vi "Main.vi"(11 "Module Admin":refnum<class "Delacor_lib_QMH_Module Admin.lvclass">) -> ()   [LabVIEW 2021, in "Host Interpreter.lvlib"]
doc: "This template is based off of the Queued Message Handler design pattern and the Queued Message Handler project template that ships with LabVIEW.\n\nThe main difference is that the queue is private to this module and communication between modules is performed via Broadcast and Request events.\n\nRequest events are wrapped in public API methods and are handled in the Event Handling Loop (EHL) of this VI. Any module can register for Broadcast events sent by this module. The EHL generates messages based on user interface actions.\n\nThe Message Handling Loop (MHL) processes messages generated by the EHL, or by other messages. The messages are string values, so new messages can be added easily to the Message Cases case structure in the MHL. Each message cluster can also provide an optional value for Message Data, which is a variant that can be converted to whatever message-specific data is required.\n_____\nBased on DQMH Dev Tools: Project Template 7.1.2.1547."
uses:
  Host Interpreter.lvlib
  <vilib>/Delacor/Delacor QMH/Libraries/Module Admin_class/Delacor_lib_QMH_Module Admin.lvclass
  Module Data--cluster.ctl
  Host Initialization--cluster.ctl
  Read Messages from Target HL--cluster.ctl
  Stop Argument--cluster.ctl
  <vilib>/Delacor/Delacor QMH/Libraries/Message Queue_class/Delacor_lib_QMH_Message Queue.lvclass/Delacor_lib_QMH_Message Queue.ctl
  <vilib>/Delacor/Delacor QMH/Libraries/Module Admin_class/Delacor_lib_QMH_Module Admin.lvclass/Delacor_lib_QMH_Module Admin.ctl
  Open UDP Argument--cluster.ctl
  Send Message to Target Argument--cluster.ctl
  Libraries/UDP Comms/UDP Message--cluster.ctl
  Close UDP Argument--cluster.ctl
  Disconnect from Target Argument--cluster.ctl
  Connected to Target Argument--cluster.ctl
  Disconnected from Target Argument--cluster.ctl
  <vilib>/Utility/miscctls.llb/LVPointTypeDef.ctl
  cda96e32-a3c6-4f37-bbf6-85d7dab5b00d.vi
  b5302b80-1133-4ea9-a211-fc2c65372a7a.vi
  1aab31dc-b2c4-46e6-995f-f9a1faaff8ea.vi
  <vilib>/Delacor/Delacor QMH/Libraries/Message Queue_class/Delacor_lib_QMH_Enqueue Message (Single).vi
  <vilib>/Delacor/Delacor QMH/Libraries/Module Admin_class/Delacor_lib_QMH_Get External Launch.vi
  <vilib>/JDP Science/JSONtext/JSON text to Variant.vi
  <vilib>/JDP Science/JSONtext/LVClass Serializer/JSONtext LVClass Serializer.lvclass
  <vilib>/Delacor/Delacor QMH/Libraries/Message Queue_class/Delacor_lib_QMH_Message Queue.lvclass
  Libraries/UDP Comms/UDP Comms.lvlib
  Libraries/Utilities/Utilities.lvlib
  Main HMI/Main HMI.lvlib
panel:
  out "error out":errorcluster
  out "Status":string
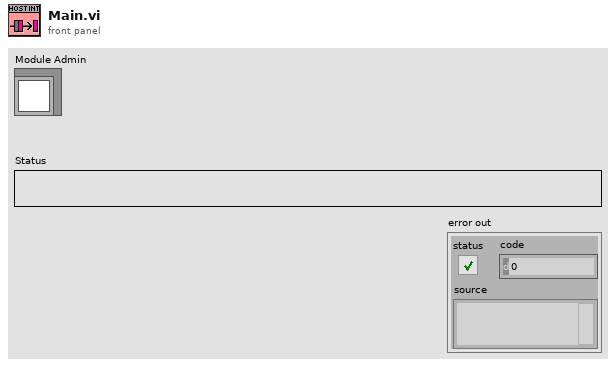
[diagram p1: front panel]
types:
  T1 = typedef "Host Interpreter.lvlib/Request Events--cluster.ctl" = cluster{"Stop Module":refnum<user-event>, "Show Panel":refnum<user-event>, "Hide Panel":refnum<user-event>, "Get Module Execution Status":refnum<user-event>, "Show Diagram":refnum<user-event>, "Connect to Target":refnum<user-event>, "Private.Get Config":refnum<user-event>, "Private.Open UDP":refnum<user-event>, "Private.Start Reading MSGs":refnum<user-event>, "Private.Send Message to Target":refnum<user-event>, "Request Connections to Target":refnum<user-event>, "Private.Close UDP":refnum<user-event>, "Update Polling Time":refnum<user-event>, "Disconnect from Target":refnum<user-event>, "Private.Connected to Target":refnum<user-event>, "Private.Disconnected from Target":refnum<user-event>}
  T2 = typedef "Host Interpreter.lvlib/Read Messages from Target HL--cluster.ctl" = cluster{"Host UDP connection ref":refnum<k16>, "Target IP":string, "Target UDP Listening Port":u16}
  T3 = typedef "Host Interpreter.lvlib/Module Data--cluster.ctl" = cluster{"Status":string, "Host UDP connection ref":refnum<k16>, "Target IP":string, "Target UDP Listening Port":u16, "Host Config":T4, "Polling Rate (ms)":i32, "UDP Connected?":bool, "Connected to Target?":bool}
  T4 = typedef "UDP Comms.lvlib/Host Initialization--cluster.ctl" = cluster{"Host IP":string, "Host Listening Port":u16, "MasterHost?":bool}
  T5 = enum32{"invalid lock state", "Not Locked", "Locked (No Password)", "Password-protected"}
  T6 = typedef "Host Interpreter.lvlib/Stop Argument--cluster.ctl" = cluster{"Origin":string, "Exit via Stop Module Req?":bool, "Wait for Module to stop?":bool}
  T7 = typedef "Host Interpreter.lvlib/Open UDP Argument--cluster.ctl" = cluster{"Boolean":bool}
  T8 = typedef "Host Interpreter.lvlib/Send Message to Target Argument--cluster.ctl" = cluster{"First Message?":bool, "UDP Message":T9}
  T9 = typedef "UDP Comms.lvlib/UDP Message--cluster.ctl" = cluster{"Command":string, "Data":variant}
  T10 = typedef "Host Interpreter.lvlib/Close UDP Argument--cluster.ctl" = cluster{"Boolean":bool}
  T11 = typedef "Host Interpreter.lvlib/Disconnect from Target Argument--cluster.ctl" = cluster{"Boolean":bool}
  T12 = typedef "Host Interpreter.lvlib/Connected to Target Argument--cluster.ctl" = cluster{"Boolean":bool}
  T13 = typedef "Host Interpreter.lvlib/Disconnected from Target Argument--cluster.ctl" = cluster{"Boolean":bool}
  T14 = typedef "LVPointTypeDef.ctl" = cluster{"Horizontal":i16, "Vertical":i16}
  T15 = enum32{"Invalid", "Standard", "Closed", "Hidden", "Minimized", "Maximized"}
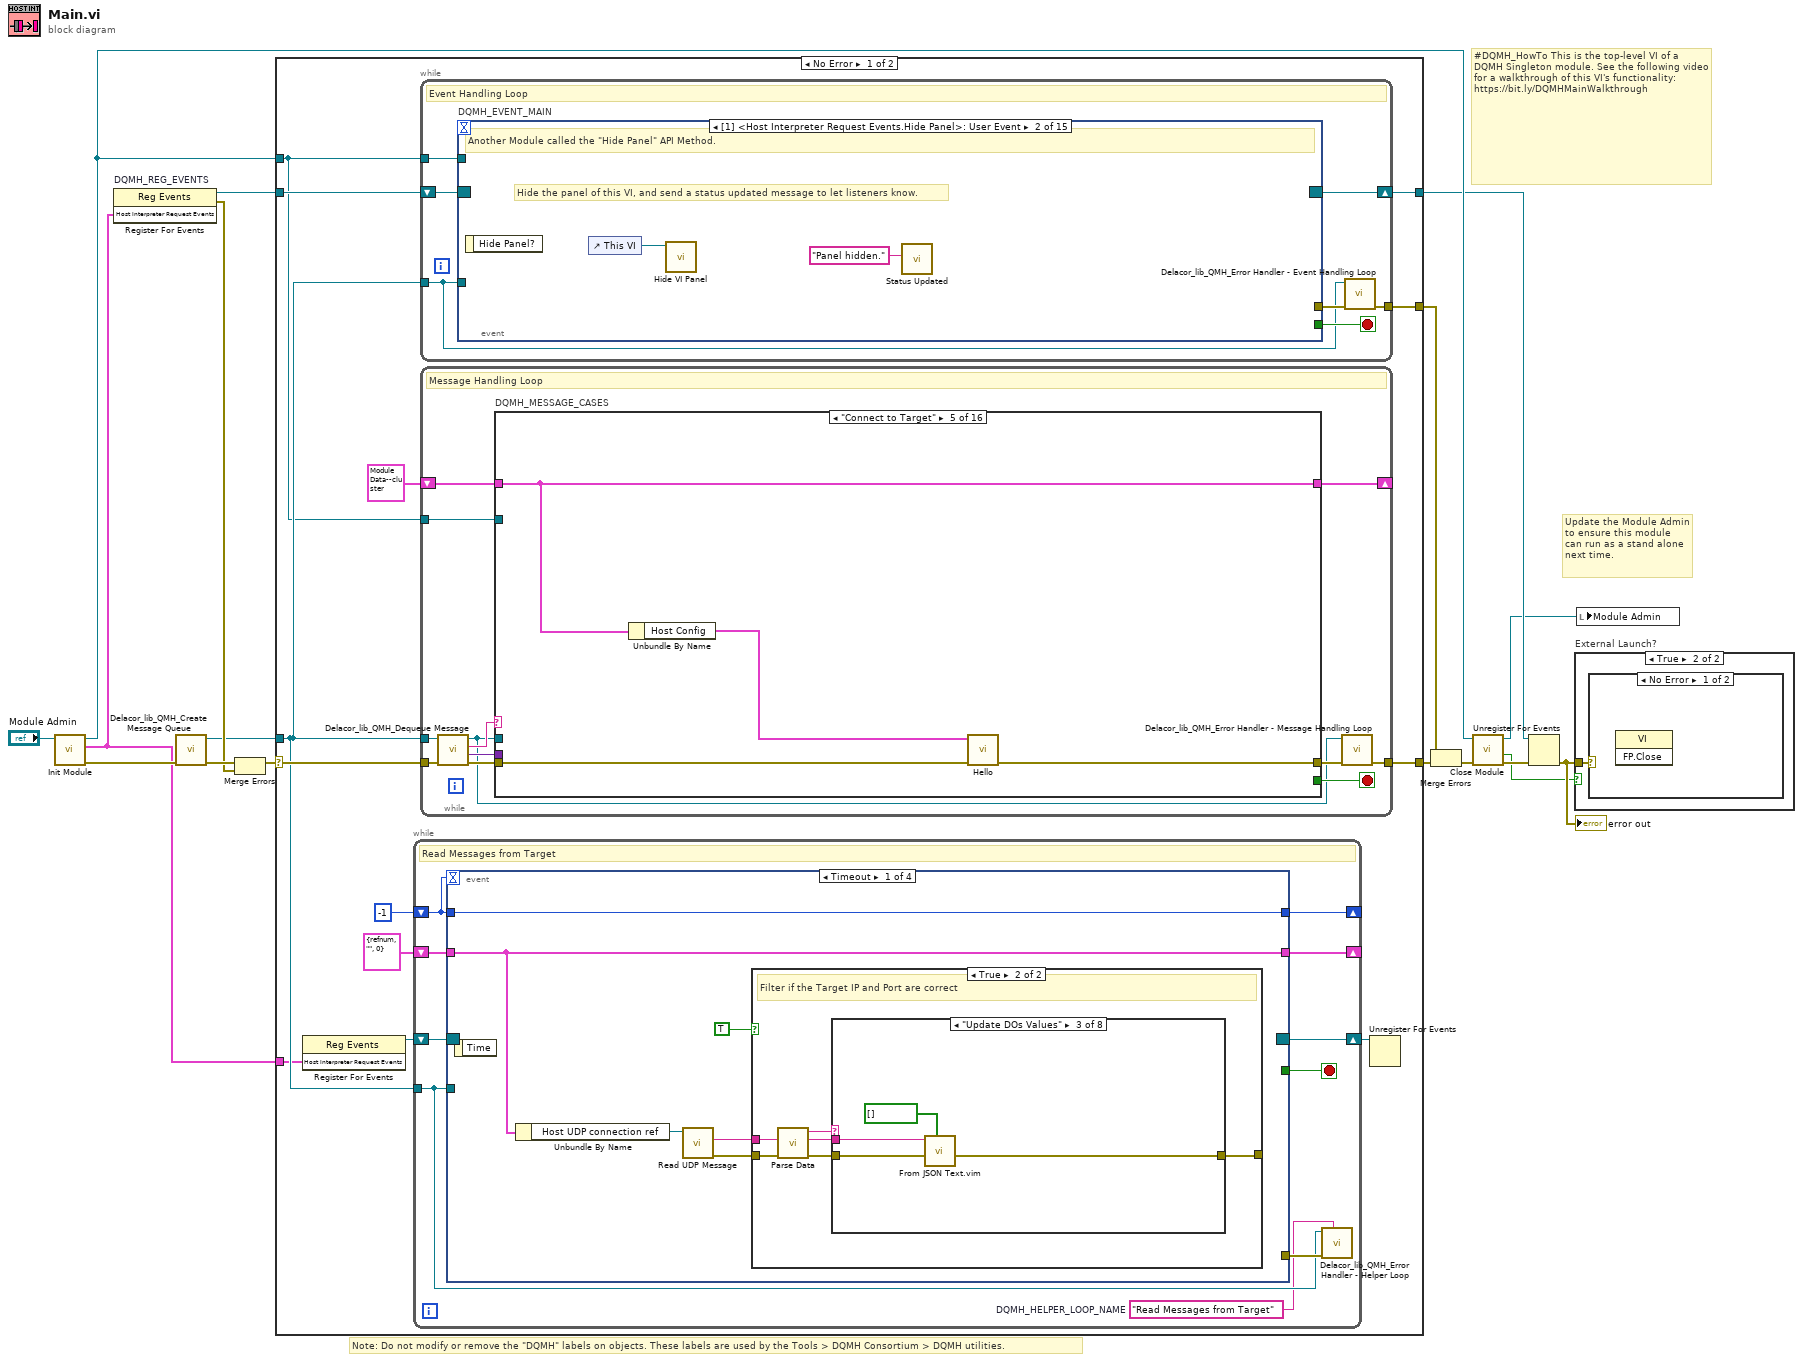
[diagram p0: block diagram]
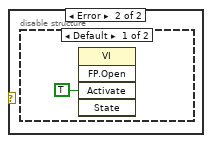
[diagram p3: hidden frame]
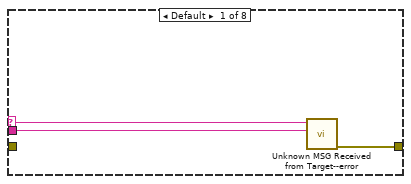
[diagram p6: hidden frame]
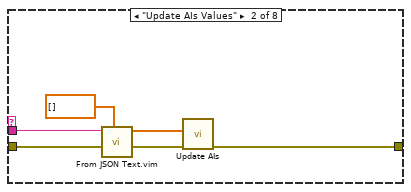
[diagram p7: hidden frame]
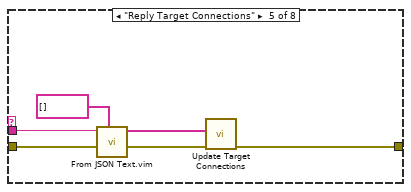
[diagram p9: hidden frame]
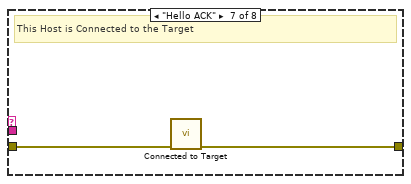
[diagram p11: hidden frame]
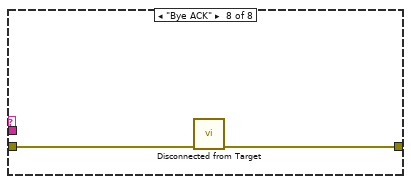
[diagram p12: hidden frame]
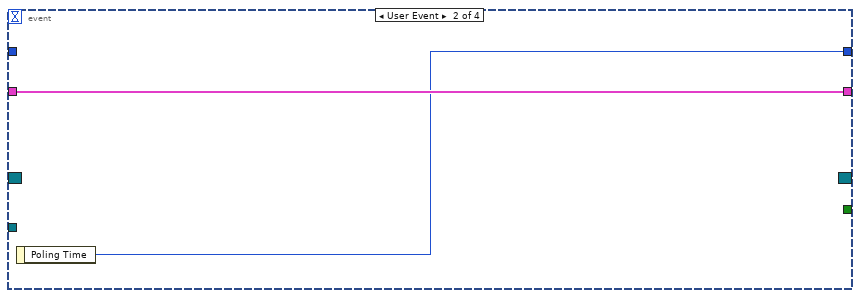
[diagram p13: hidden frame]
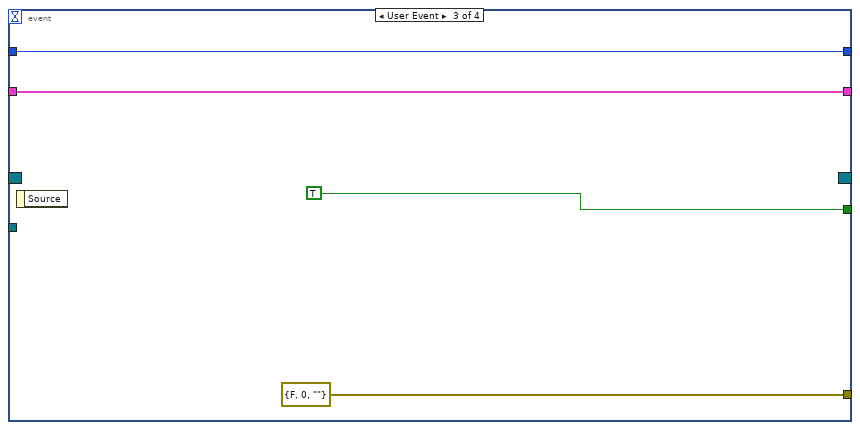
[diagram p14: hidden frame]
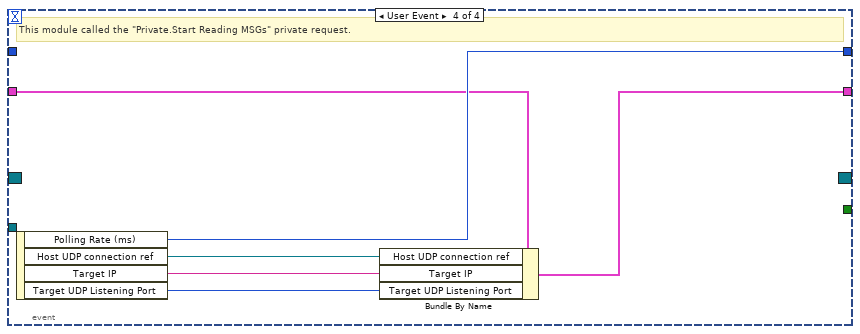
[diagram p15: hidden frame]
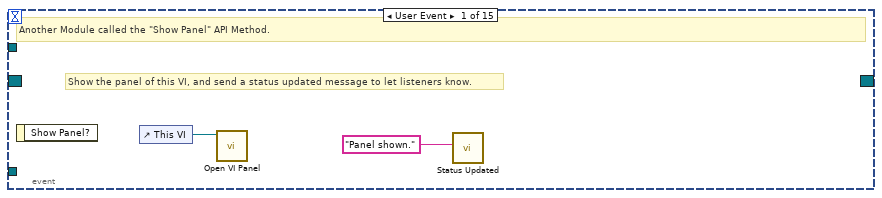
[diagram p16: hidden frame]
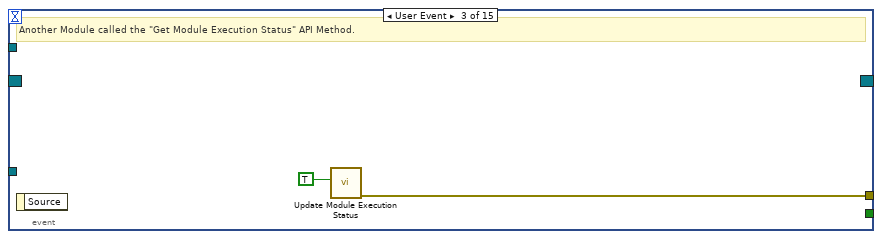
[diagram p17: hidden frame]
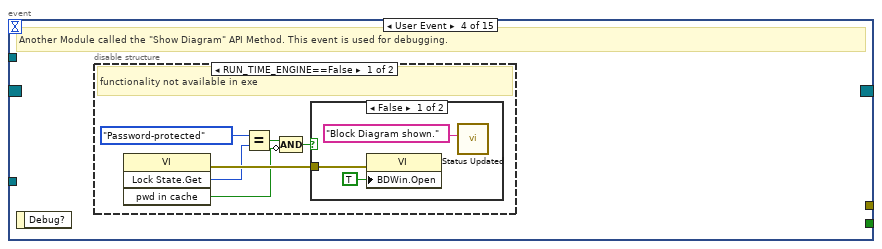
[diagram p18: hidden frame]
diagram:
  # "#DQMH_HowTo This is the top-level VI of a DQMH Singleton module. See the following video for a walkthrough of this VI's functionality: https://bit.ly/DQMHMainWalkthrough"
  # "Note: Do not modify or remove the \"DQMH\" labels on objects. These labels are used by the Tools > DQMH Consortium > DQMH utilities."
  # "Update the Module Admin to ensure this module can run as a stand alone next time."
  n1 = call "Init Module.vi"("Singleton Module Admin in"="Module Admin") -> ("error out"=w16:errorcluster, "Host Interpreter Request Events"=w1:T1, "Singleton Module Admin out"=w8:refnum<class "Delacor_lib_QMH_Module Admin.lvclass">)  [unwired: 8 in]
  n2 = register-events "DQMH_REG_EVENTS"(w1) -> (reference out=w6:refnum<event-registration>, error out=w9:errorcluster)  [unwired: 2 in]
  n3 = call <vilib>:"Delacor_lib_QMH_Create Message Queue.vi"("error in"=w16) -> ("error out"=w11:errorcluster, "Message Queue"=w5:refnum<class "Delacor_lib_QMH_Message Queue.lvclass">)  [unwired: 9 in]
  n4 = Merge Errors(w11, w9) -> (w10:errorcluster)
  n5 = case shown="No Error" w10 {
    selector: w10 -> [w28 w342]
    tunnel: [w30 w341] -> w17
    tunnel: [w27 w340] -> w7
    tunnel: w6 -> [w25 w340]
    tunnel: w5 -> [w24 w335]
    tunnel: [w29 _] -> w14
    tunnel: w8 -> [w23 w336]
    tunnel: w1 -> [w22 _]
    frame No Error {
      n6 = register-events ("DQMH_HELPER_REGFOREVENTS")(w22) -> (reference out=w20:refnum<event-registration>)  [unwired: 2 in, 1 out]
      n7 = while "DQMH_HELPER_LOOP" {
        shift-right: [w40] -> _
        shift-left: -1 -> [w39]
        shift-right: [w37] -> w21
        shift-left: w20 -> [w38]
        tunnel: w24 -> [w34]
        shift-right: [w32] -> _
        shift-left: T2 {"Host UDP connection ref"=refnum, "Target IP"="", "Target UDP Listening Port"=0} ("Read Messages from Target HL--cluster") -> [w31]
        stop <- w36 stop-if-true
        w33 = "Read Messages from Target"  # DQMH_HELPER_LOOP_NAME
        # "Read Messages from Target"
        n8 = event "DQMH_HELPER_EVENT_STRUCTURE" shown="[0] Timeout" {
          selector: w38 -> [_ _ _ _]
          dyn-events: [_ _ _ _] -> w37
          timeout: w39 -> [_ _ _ _]
          tunnel: w39 -> [w46 _ w84 _]
          tunnel: [w46 w79 w84 w90] -> w40
          tunnel: [_ _ TRUE _] -> w36
          tunnel: [_ _ errorcluster {"status"=FALSE, "code"=0, "source"=""} ("error constant") _] -> w35
          tunnel: w34 -> [_ _ _ _]
          tunnel: [w45 w80 w81 w88] -> w32
          tunnel: w31 -> [w45 w80 w81 w89]
          event Timeout {
            n9 = event-data() -> ()  [unwired: 1 in, 1 out]
            n10 = Unbundle By Name(w45) -> ("Host UDP connection ref"=w41:refnum<k16>)
            n11 = call "Read UDP Message.vi"("Local UDP connection ref"=w41) -> ("error out"=w44:errorcluster, "data out"=w43:string)  [unwired: 6 in, 3 out]
            n12 = case shown="True" TRUE {
              tunnel: w44 -> [w47 w53]
              tunnel: w43 -> [_ w52]
              tunnel: [w47 w48] -> _
              frame False {
              }
              frame True {
                # "Filter if the Target IP and Port are correct"
                n13 = call "Parse Data.vi"("error in (no error)"=w53, "Received UDP Data"=w52) -> ("error out"=w50:errorcluster, "Data"=w49:string, "Command"=w51:string)  [unwired: 7 in]
                n14 = case shown="\"Update DOs Values\"" w51 {
                  selector: w51 -> [w55 _ _ _ _ _ _ _]
                  tunnel: w50 -> [_ w62 w65 w67 w73 w74 w76 w78]
                  tunnel: w49 -> [w54 w61 w64 _ w72 _ _ _]
                  tunnel: [w56 w57 w63 w67 w69 w74 w75 w77] -> w48
                  frame Default {
                    n15 = call "Unknown MSG Received from Target--error.vi"("Data"=w54, "Command"=w55) -> ("error out"=w56:errorcluster)  [unwired: 9 in]
                  }
                  frame "Update AIs Values" {
                    n16 = call "From JSON Text.vim"("Data Type and Default Value"=dbl[] [], "error in (no error)"=w62, "JSON"=w61) -> ("error out"=w59:errorcluster, "Data out"=w58:dbl[])  [unwired: 7 in]
                    n17 = call "Update AIs.vi"("error in"=w59, "AI Values"=w58) -> ("error out"=w57:errorcluster)  [unwired: 9 in]
                  }
                  frame "Update DOs Values" {
                    n18 = call "From JSON Text.vim"("Data Type and Default Value"=bool[] [], "error in (no error)"=w65, "JSON"=w64) -> ("error out"=w63:errorcluster)  [unwired: 7 in, 1 out]
                  }
                  frame "--- Reply MSGS ---" {
                  }
                  frame "Reply Target Connections" {
                    n19 = call "From JSON Text.vim"("Data Type and Default Value"=string[] [], "error in (no error)"=w73, "JSON"=w72) -> ("error out"=w70:errorcluster, "Data out"=w68:string[])  [unwired: 7 in]
                    n20 = call "Update Target Connections.vi"("error in"=w70, "Target Connections"=w68) -> ("error out"=w69:errorcluster)  [unwired: 9 in]
                  }
                  frame "--- ACK MSGs ---" {
                  }
                  frame "Hello ACK" {
                    # "This Host is Connected to the Target"
                    n21 = call "Connected to Target.vi"("error in"=w76) -> ("error out"=w75:errorcluster)  [unwired: 10 in]
                  }
                  frame "Bye ACK" {
                    n22 = call "Disconnected from Target.vi"("error in"=w78) -> ("error out"=w77:errorcluster)  [unwired: 10 in]
                  }
                }
              }
            }
          }
          event User Event {
            n23 = event-data() -> ("Poling Time"=w79:i32)  [unwired: 1 in]
          }
          event User Event {
            n24 = event-data() -> ()  [unwired: 1 in, 1 out]
          }
          event User Event {
            # "This module called the \"Private.Start Reading MSGs\" private request."
            n25 = event-data() -> ("Polling Rate (ms)"=w90:i32, "Host UDP connection ref"=w87:refnum<k16>, "Target IP"=w86:string, "Target UDP Listening Port"=w85:u16)  [unwired: 1 in]
            n26 = Bundle By Name(cluster=w89, "Host UDP connection ref"=w87, "Target IP"=w86, "Target UDP Listening Port"=w85) -> (w88:T2)
          }
        }
        n27 = call-dynamic "Delacor_lib_QMH_Error Handler - Helper Loop.vi"("Error Debug"=w33, "error in"=w35, "Message Queue in"=w34) -> ()  [unwired: 7 in, 2 out]
      }
      n28 = while {
        tunnel: w24 -> [w91]
        shift-right: [w94] -> w27
        shift-left: w25 -> [w95]
        tunnel: [w96] -> w29
        tunnel: w23 -> [w92]
        stop <- w93 stop-if-true
        # "Event Handling Loop"
        n29 = event "DQMH_EVENT_MAIN" shown="[1] <Host Interpreter Request Events.Hide Panel>: User Event" {
          selector: w95 -> [_ _ _ _ _ _ _ _ _ _ _ _ _ _ _]
          dyn-events: [_ _ _ _ _ _ _ _ _ _ _ _ _ _ _] -> w94
          timeout: _ -> [_ _ _ _ _ _ _ _ _ _ _ _ _ _ _]
          tunnel: [_ _ _ _ TRUE ("Discard?") _ _ _ _ _ _ _ _ _ _] -> w93
          tunnel: w91 -> [_ _ _ _ w120 w127 w139 w142 w148 w155 w158 w164 w170 w176 w182]
          tunnel: [_ _ w103 _ w123 w129 w137 w140 w143 w151 w156 w159 w165 w171 w177] -> w97
          tunnel: w92 -> [_ _ _ _ _ w126 _ _ _ _ _ _ _ _ _]
          event User Event {
            # "Show the panel of this VI, and send a status updated message to let listeners know."
            # "Another Module called the \"Show Panel\" API Method."
            n30 = event-data() -> ()  [unwired: 1 in, 1 out]
            n31 = control-ref of="This VI"() -> (w99:refnum<vi>)
            n32 = call "Open VI Panel.vi"("VI"=w99) -> ()  [unwired: 10 in, 1 out]
            n33 = call "Status Updated.vi"("Status"="Panel shown." ("format string")) -> ()  [unwired: 10 in, 1 out]
          }
          event User Event {
            # "Hide the panel of this VI, and send a status updated message to let listeners know."
            # "Another Module called the \"Hide Panel\" API Method."
            n34 = event-data() -> ()  [unwired: 1 in, 1 out]
            n35 = control-ref of="This VI"() -> (w101:refnum<vi>)
            n36 = call "Hide VI Panel.vi"("VI"=w101) -> ()  [unwired: 10 in, 1 out]
            n37 = call "Status Updated.vi"("Status"="Panel hidden." ("format string")) -> ()  [unwired: 10 in, 1 out]
          }
          event User Event {
            # "Another Module called the \"Get Module Execution Status\" API Method."
            n38 = event-data() -> ()  [unwired: 1 in, 1 out]
            n39 = call "Update Module Execution Status.vi"("Running?"=TRUE) -> ("error out"=w103:errorcluster)  [unwired: 10 in]
          }
          event User Event {
            # "Another Module called the \"Show Diagram\" API Method. This event is used for debugging."
            n40 = event-data() -> ()  [unwired: 1 in, 1 out]
            n41 = disable-structure shown="RUN_TIME_ENGINE==False" {
              frame condition #0 (active) {
                # "functionality not available in exe"
                n42 = invoke on="Invoke Node" class="VI" method="Lock State.Get"() -> (error out=w109:errorcluster, "Get Lock State"=w108:T5, "pwd in cache"=w105:bool)  [unwired: 4 in, 1 out]
                n43 = Equal?(x=T5."Password-protected", y=w108) -> (x = y?=w106:bool)
                n44 = Compound Arithmetic op=AND(w106, invert w105) -> (w104:bool)
                n45 = case shown="False" w104 {
                  tunnel: w109 -> [w112 _]
                  frame False {
                    n46 = property on="Property Node" class="VI"(error in=w112, "BDWin.Open"=TRUE ("Block Diagram Window:Open")) -> ()  [unwired: 1 in, 2 out]
                    n47 = call "Status Updated.vi"("Status"="Block Diagram shown." ("format string")) -> ()  [unwired: 10 in, 1 out]
                  }
                  frame True {
                    # "Password-protected VI, and the password is not in the cache. Do not show the diagram."
                  }
                }
              }
              frame condition #1 {
              }
            }
          }
          event User Event {
            # "The Stop Module Event can get fired from the Exit message in the MHL. The queue gets destroyed in that case. If the queue no longer exists, the Enqueue Exit as a priority message will return error 1. It is safe to ignore, because the module is already exiting."
            # "Another Module called the \"Stop Module\" API Method  or the Message Handling Loop below."
            n48 = event-data() -> ("Origin"=w119:string, "Exit via Stop Module Req?"=w115:bool, "Wait for Module to stop?"=w114:bool)  [unwired: 1 in]
            n49 = local write "Status"(w119) -> ()
            n50 = Bundle By Name(cluster=T6 {"Origin"="", "Exit via Stop Module Req?"=FALSE, "Wait for Module to stop?"=FALSE} ("Stop Argument"), "Exit via Stop Module Req?"=w115, "Wait for Module to stop?"=w114) -> (w113:T6)
            n51 = call-poly <vilib>:"Delacor_lib_QMH_Enqueue Message (poly).vi"("Priority Message? (F)"=TRUE, "Message Data"=w113, "Message"="Exit", "Message Queue in"=w120) -> ("error out"=w124:errorcluster)  [unwired: 6 in, 1 out]
            n52 = call <vilib>:"Clear Errors.vi"("error in (no error)"=w124, "specific error code to clear (0: all)"=1) -> ("error out"=w123:errorcluster)  [unwired: 4 in, 1 out]
          }
          event Panel Close? {
            w128 = TRUE  # Discard the event, the MHL is responsible for closing and stopping this VI.
            # "Hide the panel or send the 'Exit' message if the user clicks the 'X' on the module main VI panel."
            n53 = event-data() -> ()  [unwired: 1 in, 1 out]
            n54 = property on="Property Node" class="Module Admin"(reference=w126) -> ("Accessors:External Launch"=w125:bool)  [unwired: 1 in, 2 out]
            n55 = case shown="True" w125 {
              tunnel: w127 -> [_ w135]
              tunnel: [_ w136] -> w129
              frame True {
                # "If externally launched, clicking the 'X' hides the panel, but doesn't close it."
                n56 = control-ref of="This VI"() -> (w132:refnum<vi>)
                n57 = call "Hide VI Panel.vi"("VI"=w132) -> ("error out"=w130:errorcluster)  [unwired: 10 in]
                n58 = call "Status Updated.vi"("error in"=w130, "Status"="Panel hidden." ("format string")) -> ()  [unwired: 9 in, 1 out]
              }
              frame False {
                # "If run as a stand-alone VI, clicking the panel 'X' stops the VI."
                n59 = call-poly <vilib>:"Delacor_lib_QMH_Enqueue Message (poly).vi"("Priority Message? (F)"=TRUE, "Message"="Exit", "Message Queue in"=w135) -> ("error out"=w136:errorcluster)  [unwired: 7 in, 1 out]
              }
            }
            n60 = event-data ("Event Filter Node")("Discard?"=w128) -> ()  [unwired: 1 in, 1 out]
          }
          event User Event {
            # "Another Module called the \"Connect to Target\" API Method."
            n61 = event-data() -> ()  [unwired: 1 in, 1 out]
            n62 = call-poly <vilib>:"Delacor_lib_QMH_Enqueue Message (poly).vi"("Message"="Connect to Target", "Message Queue in"=w139) -> ("error out"=w137:errorcluster)  [unwired: 8 in, 1 out]
          }
          event User Event {
            # "This module called the \"Private.Get Config\" private request."
            n63 = event-data() -> ()  [unwired: 1 in, 1 out]
            n64 = call-poly <vilib>:"Delacor_lib_QMH_Enqueue Message (poly).vi"("Message"="Get Config", "Message Queue in"=w142) -> ("error out"=w140:errorcluster)  [unwired: 8 in, 1 out]
          }
          event User Event {
            # "This module called the \"Private.Open UDP\" private request."
            n65 = event-data() -> ("Boolean"=w144:bool)  [unwired: 1 in]
            n66 = Bundle(cluster=T7 {"Boolean"=FALSE} ("Open UDP Argument"), "Boolean"=w144) -> (w145:T7)
            n67 = call-poly <vilib>:"Delacor_lib_QMH_Enqueue Message (poly).vi"("Message Data"=w145, "Message"="Open UDP", "Message Queue in"=w148) -> ("error out"=w143:errorcluster)  [unwired: 7 in, 1 out]
          }
          event User Event {
            # "This module called the \"Private.Send Message to Target\" private request."
            n68 = event-data() -> ("First Message?"=w149:bool, "UDP Message"=w150:T9)  [unwired: 1 in]
            n69 = Bundle(cluster=T8 {"First Message?"=FALSE, "UDP Message"={"Command"="", "Data"=variant}} ("Send Message to Target Argument"), "First Message?"=w149, "UDP Message"=w150) -> (w152:T8)
            n70 = call-poly <vilib>:"Delacor_lib_QMH_Enqueue Message (poly).vi"("Message Data"=w152, "Message"="Send Message to Target", "Message Queue in"=w155) -> ("error out"=w151:errorcluster)  [unwired: 7 in, 1 out]
          }
          event User Event {
            # "Another Module called the \"Request Connections to Target\" API Method."
            n71 = event-data() -> ()  [unwired: 1 in, 1 out]
            n72 = call-poly <vilib>:"Delacor_lib_QMH_Enqueue Message (poly).vi"("Message"="Request Connections to Target", "Message Queue in"=w158) -> ("error out"=w156:errorcluster)  [unwired: 8 in, 1 out]
          }
          event User Event {
            # "This module called the \"Private.Close UDP\" private request."
            n73 = event-data() -> ("Boolean"=w160:bool)  [unwired: 1 in]
            n74 = Bundle(cluster=T10 {"Boolean"=FALSE} ("Close UDP Argument"), "Boolean"=w160) -> (w161:T10)
            n75 = call-poly <vilib>:"Delacor_lib_QMH_Enqueue Message (poly).vi"("Message Data"=w161, "Message"="Close UDP", "Message Queue in"=w164) -> ("error out"=w159:errorcluster)  [unwired: 7 in, 1 out]
          }
          event User Event {
            # "Another Module called the \"Disconnect from Target\" API Method."
            n76 = event-data() -> ("Boolean"=w166:bool)  [unwired: 1 in]
            n77 = Bundle(cluster=T11 {"Boolean"=FALSE} ("Disconnect from Target Argument"), "Boolean"=w166) -> (w167:T11)
            n78 = call-poly <vilib>:"Delacor_lib_QMH_Enqueue Message (poly).vi"("Message Data"=w167, "Message"="Disconnect from Target", "Message Queue in"=w170) -> ("error out"=w165:errorcluster)  [unwired: 7 in, 1 out]
          }
          event User Event {
            # "This module called the \"Private.Connected to Target\" private request."
            n79 = event-data() -> ("Boolean"=w172:bool)  [unwired: 1 in]
            n80 = Bundle(cluster=T12 {"Boolean"=FALSE} ("Connected to Target Argument"), "Boolean"=w172) -> (w173:T12)
            n81 = call-poly <vilib>:"Delacor_lib_QMH_Enqueue Message (poly).vi"("Message Data"=w173, "Message"="Connected to Target", "Message Queue in"=w176) -> ("error out"=w171:errorcluster)  [unwired: 7 in, 1 out]
          }
          event User Event {
            # "This module called the \"Private.Disconnected from Target\" private request."
            n82 = event-data() -> ("Boolean"=w178:bool)  [unwired: 1 in]
            n83 = Bundle(cluster=T13 {"Boolean"=FALSE} ("Disconnected from Target Argument"), "Boolean"=w178) -> (w179:T13)
            n84 = call-poly <vilib>:"Delacor_lib_QMH_Enqueue Message (poly).vi"("Message Data"=w179, "Message"="Disconnected from Target", "Message Queue in"=w182) -> ("error out"=w177:errorcluster)  [unwired: 7 in, 1 out]
          }
        }
        n85 = call-dynamic "Delacor_lib_QMH_Error Handler - Event Handling Loop.vi"("error in"=w97, "Message Queue in"=w91) -> ("dup error in"=w96:errorcluster)  [unwired: 8 in, 1 out]
      }
      n86 = while {
        tunnel: w24 -> [w183]
        shift-right: [w191] -> _
        shift-left: T3 {"Status"="", "Host UDP connection ref"=refnum, "Target IP"="", "Target UDP Listening Port"=0, "Host Config"={"Host IP"="", "Host Listening Port"=0, "MasterHost?"=FALSE}, "Polling Rate (ms)"=-1, "UDP Connected?"=FALSE, "Connected to Target?"=FALSE} ("Data Cluster") -> [w192]
        tunnel: w28 -> [w194]
        tunnel: [w186] -> w30
        tunnel: w23 -> [w187]
        stop <- w190 stop-if-true
        # "Message Handling Loop"
        n87 = call-dynamic "Delacor_lib_QMH_Dequeue Message.vi"("error in"=w194, "Message Queue in"=w183) -> ("error out"=w193:errorcluster, "Message Data"=w188:variant, "Message"=w189:string, "Message Queue out"=w184:refnum<class "Delacor_lib_QMH_Message Queue.lvclass">)  [unwired: 6 in]
        n88 = case "DQMH_MESSAGE_CASES" shown="\"Connect to Target\"" w189 {
          selector: w189 -> [_ _ _ _ _ _ _ _ _ _ _ _ _ _ _ w330]
          tunnel: w184 -> [_ _ _ _ _ _ _ _ _ _ _ _ _ w295 w318 _]
          tunnel: w193 -> [w212 w216 w219 w239 w242 w250 w267 w269 w276 w281 w285 w289 w291 w302 w324 w333]
          tunnel: [w210 w216 w218 w232 w241 w253 w266 w272 w275 w279 w285 w288 w291 w298 w319 w334] -> w185
          tunnel: w192 -> [w201 w215 w226 w238 w243 w252 w268 w271 w274 w282 w286 w287 w290 w297 w310 w331]
          tunnel: [w200 w215 w225 w234 w243 w252 w268 w271 w274 w278 w284 w287 w290 w297 w310 w331] -> w191
          tunnel: [_ _ _ _ _ _ _ _ _ _ _ _ _ _ w317 _] -> w190
          tunnel: w188 -> [_ _ _ _ _ w249 _ _ _ _ _ _ _ w296 w316 _]
          tunnel: w187 -> [w202 _ _ _ _ _ _ _ _ _ _ _ _ w294 w311 _]
          frame "Initialize" {
            w196 = "Initial Message" ("Initial Message")
            # "Initialize - Any operation that needs to be done before the module can receive messages. Synchronize Caller Events.vi will inform Start Module.vi that the module has launched and is ready to receive messages. Module Did Init.vi will broadcast that the module initialized."
            n89 = call "Synchronize Caller Events.vi"("error in"=w212, "Singleton Module Admin in"=w202) -> ("error out"=w211:errorcluster, "Singleton Module Admin out"=w197:refnum<class "Delacor_lib_QMH_Module Admin.lvclass">)  [unwired: 8 in]
            n90 = property on="Property Node" class="Module Admin"(reference=w197) -> ("Accessors:External Launch"=w206:bool)  [unwired: 1 in, 2 out]
            n91 = Select(t=T15."Hidden" ("State"), s=w206, f=T15."Standard" ("State")) -> (s? t:f=w203:T15)
            n92 = call "Module Name--constant.vi"() -> ("Module Name"=w209:string)  [unwired: 11 in]
            n93 = property on="Property Node" class="VI"("Front Panel.Title"=w209) -> (reference out=w208:refnum<vi>, error out=w214:errorcluster)  [unwired: 2 in]
            n94 = invoke on="Invoke Node" class="VI" method="FP.Open"(reference=w208, error in=w214, "State"=w203) -> (reference out=w207:refnum<vi>, error out=w213:errorcluster)  [unwired: 2 in, 3 out]
            n95 = Bundle By Name(cluster=w201, "Status"=w196) -> (w200:T3)
            n96 = call "Get Config.vi"() -> ()  [unwired: 11 in, 1 out]
            n97 = invoke on="Invoke Node" class="VI" method="FP.Center"(reference=w207, error in=w213) -> ()  [unwired: 1 in, 3 out]
            n98 = property on="Pane" class="Pane"("Origin"=T14 {"Horizontal"=0, "Vertical"=0}) -> ()  [unwired: 2 in, 2 out]
            n99 = call "Module Name--constant.vi"() -> ("Module Name"=w198:string)  [unwired: 11 in]
            n100 = call "Module Did Init.vi"("error in"=w211, "Initialized?"=TRUE, "Origin"=w198) -> ("error out"=w210:errorcluster)  [unwired: 8 in]
            "Status" <- w196
          }
          frame "---Module Specific---" {
            # "Separator -- The following cases handle messages specific to this Module."
          }
          frame "Get Config" {
            n101 = call "Get Local IP.vi"() -> ("Local IP"=w222:string)  [unwired: 4 in]
            n102 = Bundle By Name(cluster=w226, "Host Config.Host IP"=w222, "Host Config.Host Listening Port"=u16 12390, "Host Config.MasterHost?"=TRUE, "Target UDP Listening Port"=u16 61670 ("Port RT"), "Target IP"="192.168.1.163" ("IP RT"), "Polling Rate (ms)"=1000 ("Polling Rate")) -> (w225:T3)
            n103 = call "Open UDP.vi"("error in"=w219) -> ("error out"=w218:errorcluster)  [unwired: 10 in]
          }
          frame "Open UDP" {
            n104 = Unbundle By Name(w238) -> ("Polling Rate (ms)"=w228:i32, "Target UDP Listening Port"=w230:u16, "Target IP"=w229:string, "Host Config.Host IP"=w236:string, "Host Config.Host Listening Port"=w237:u16)
            n105 = String To IP(1:w236) -> (0:w235:u32)
            n106 = UDP Open(7:w235, 8:w239, 11:w237) -> (port=w231:refnum<k16>, 0:w233:errorcluster)  [unwired: 2 in, 1 out]
            n107 = Bundle By Name(cluster=w238, "UDP Connected?"=TRUE, "Host UDP connection ref"=w231) -> (w234:T3)
            n108 = call "Start Reading MSGs.vi"("Polling Rate (ms)"=w228, "Target IP"=w229, "Target UDP Listening Port"=w230, "Host UDP connection ref"=w231) -> ()  [unwired: 7 in, 1 out]
            n109 = call "Connect to Target.vi"("error in"=w233) -> ("error out"=w232:errorcluster)  [unwired: 10 in]
          }
          frame "Connect to Target" {
            n110 = Unbundle By Name(w243) -> ("Host Config"=w240:T4)
            n111 = call "Hello.vi"("error in"=w242, "Host Initialization--cluster"=w240) -> ("error out"=w241:errorcluster)  [unwired: 9 in]
          }
          frame "Send Message to Target" {
            n112 = Variant To Data(error in=w250, type=T8 {"First Message?"=FALSE, "UDP Message"={"Command"="", "Data"=variant}} ("Send Message to Target Argument"), Variant=w249) -> (data=w246:T8, error out=w247:errorcluster)
            n113 = Unbundle By Name(w252) -> ("Connected to Target?"=w251:bool)
            n114 = Unbundle By Name(w246) -> ("First Message?"=w244:bool)
            n115 = Or(x=w251, y=w244) -> (x .or. y?=w245:bool)
            n116 = case shown="True" w245 {
              tunnel: w252 -> [_ w261]
              tunnel: [w254 w257] -> w253
              tunnel: w246 -> [_ w256]
              tunnel: w247 -> [_ w255]
              frame False {
                n117 = call "MSG to Target Cannot be Sent --error.vi"() -> ("error out"=w254:errorcluster)  [unwired: 11 in]
              }
              frame True {
                n118 = Unbundle By Name(w261) -> ("Target UDP Listening Port"=w258:u16, "Target IP"=w259:string, "Host UDP connection ref"=w260:refnum<k16>)
                n119 = Unbundle By Name(w256) -> ("UDP Message.Command"=w264:string, "UDP Message.Data"=w263:variant)
                n120 = call "Build Data.vi"("error in (no error)"=w255, "Data"=w263, "Command"=w264) -> ("error out"=w265:errorcluster, "UDP MSG To be Sent"=w262:string)  [unwired: 7 in]
                n121 = call "Send UDP Message.vi"("Remote UDP Listening Port"=w258, "Remote IP"=w259, "error in"=w265, "UDP Data to be sent"=w262, "Local UDP connection ref"=w260) -> ("error out"=w257:errorcluster)  [unwired: 5 in, 1 out]
              }
            }
          }
          frame "Request Connections to Target" {
            n122 = call "Request Target Connections.vi"("error in"=w267) -> ("error out"=w266:errorcluster)  [unwired: 10 in]
          }
          frame "Close UDP" {
            n123 = Unbundle By Name(w271) -> ("Host UDP connection ref"=w270:refnum<k16>)
            n124 = UDP Close(connection ID=w270, 8:w269) -> (error out=w272:errorcluster)  [unwired: 1 out]
          }
          frame "Disconnect from Target" {
            n125 = Unbundle By Name(w274) -> ("Host Config"=w273:T4)
            n126 = call "Bye.vi"("error in"=w276, "Host Initialization--cluster"=w273) -> ("error out"=w275:errorcluster)  [unwired: 9 in]
          }
          frame "Connected to Target" {
            n127 = Bundle By Name(cluster=w282, "Connected to Target?"=TRUE) -> (w278:T3)
            n128 = call "Connected.vi"("error in"=w281) -> ("error out"=w280:errorcluster)  [unwired: 10 in]
            n129 = call "Request Connections to Target.vi"("error in"=w280) -> ("error out"=w279:errorcluster)  [unwired: 10 in]
          }
          frame "Disconnected from Target" {
            n130 = Bundle By Name(cluster=w286, "Connected to Target?"=FALSE) -> (w284:T3)
            n131 = call "Disconnected.vi"() -> ()  [unwired: 11 in, 1 out]
          }
          frame "---Copy This Frame---" {
            # "Duplicate this frame when creating new messages.  Change this comment in the duplicated frame to describe this message."
            n132 = Merge Errors(w289) -> (w288:errorcluster)
          }
          frame "---Exit and Error Handling---" {
            # "Separator - The following cases handle errors and exit messages."
          }
          frame "Error" {
            # "#DQMH_CodeRecommended - If the module is running in standalone mode (External Launch = FALSE), this code will pop up an error dialog and call the 'Exit' message if an error occurs. Add more fine-grained error management here."
            # "Error - Check the error message data and respond accordingly. This message is sent by the \"Error Handler\" VIs at the end of each loop in this application."
            n133 = property on="Property Node" class="Module Admin"(reference=w294) -> ("Accessors:External Launch"=w293:bool)  [unwired: 1 in, 2 out]
            n134 = Variant To Data(error in=w302, type=errorcluster {"status"=FALSE, "code"=0, "source"=""} ("error constant"), Variant=w296) -> (data=w292:errorcluster, error out=w300:errorcluster)
            n135 = local write "error out"(w292) -> ()
            n136 = call "Error Reported.vi"("Error"=w292) -> ()  [unwired: 10 in, 1 out]
            n137 = case shown="False" w293 {
              tunnel: [w307 _] -> w299
              tunnel: w295 -> [w305 _]
              tunnel: w292 -> [w306 _]
              frame False {
                n138 = disable-structure shown="Default" {
                  disable-tunnel: w306 -> [w308 _]
                  frame condition #0 (active) {
                    # "If the module is running standalone, then pop up an error dialog and call the \"Exit\" message."
                    n139 = call <vilib>:"Simple Error Handler.vi"("error in (no error)"=w308) -> ()  [unwired: 4 in, 5 out]
                  }
                  frame condition #1 {
                    # "To prevent the Simple Error Handler VI from being loaded (e.g. when deploying to a Real-Time target), add the Conditional Disable Symbol \"DQMH_Disable_SEH\" to your project and set it to TRUE."
                  }
                }
                n140 = call-poly <vilib>:"Delacor_lib_QMH_Enqueue Message (poly).vi"("Priority Message? (F)"=TRUE, "Message"="Exit", "Message Queue in"=w305) -> ("error out"=w307:errorcluster)  [unwired: 7 in, 1 out]
              }
              frame True {
                # "If the module was launched externally, calling the Error Reported broadcast VI is the only action performed by the \"Error\" message. The module's caller can then process the error appropriately."
              }
            }
            n141 = Merge Errors(w300, w299) -> (w298:errorcluster)
          }
          frame "Exit" {
            w315 = 91  # 91: not all Exit messages will have an argument
            w317 = TRUE  # Stop the VI
            # "Release the message queue reference"
            # "#DQMH_CodeNeeded - Add any required cleanup code here."
            # "Exit - Exit the application."
            n142 = Variant To Data(error in=w324, type=T6 {"Origin"="", "Exit via Stop Module Req?"=FALSE, "Wait for Module to stop?"=FALSE} ("Stop Argument"), Variant=w316) -> (data=w313:T6, error out=w321:errorcluster)
            n143 = call <vilib>:"Clear Errors.vi"("error in (no error)"=w321, "specific error code to clear (0: all)"=w315) -> ("error out"=w323:errorcluster)  [unwired: 4 in, 1 out]
            n144 = control-ref of="This VI"() -> (w312:refnum<vi>)
            n145 = call-dynamic "Delacor_lib_QMH_Release Message Queue.vi"("error in"=w323, "Message Queue"=w318) -> ("error out"=w322:errorcluster)  [unwired: 9 in]
            n146 = call "Handle Exit.vi"("Stop Argument"=w313, "Admin in"=w311, "VI reference"=w312) -> ("error out"=w320:errorcluster)  [unwired: 7 in, 1 out]
            n147 = Merge Errors(w322, w320) -> (w319:errorcluster)
            n148 = Unbundle By Name(w310) -> ("Host UDP connection ref"=w309:refnum<k16>)
            n149 = call "Error Reported.vi"("Error"=w319) -> ()  [unwired: 10 in, 1 out]
            n150 = UDP Close(connection ID=w309) -> ()  [unwired: 1 in, 2 out]
          }
          frame Default {
            # "'Default' case only runs if there is a message that isn't defined in any of the other cases.  Output a programming error."
            n151 = call "Module Name--constant.vi"() -> ("Module Name"=w329:string)  [unwired: 11 in]
            n152 = Format Into String(format string="The invalid message string \"%s\" was received in the Message Handling Loop for module \"%s\".", w330, w329) -> (resulting string=w325:string)  [unwired: 2 in, 1 out]
            n153 = call <vilib>:"Error Cluster From Error Code.vi"("show call chain? (False)"=TRUE, "error message (\"\")"=w325, "error code (0)"=1) -> ("error out"=w332:errorcluster)  [unwired: 6 in]
            n154 = Merge Errors(w333, w332) -> (w334:errorcluster)
          }
        }
        n155 = call-dynamic "Delacor_lib_QMH_Error Handler - Message Handling Loop.vi"("error in"=w185, "Message Queue in"=w184) -> ("dup error in"=w186:errorcluster)  [unwired: 8 in, 1 out]
      }
      n156 = Unregister For Events(event registration refnum=w21) -> ()  [unwired: 1 in, 1 out]
    }
    frame Error {
      # "Synchronize Caller Events.vi will inform Start Module.vi that the module has launched and will let the code calling Start Module.vi register for broadcasts and would permit the caller receive the broadcast that an error occurred at launch time."
      n157 = call-dynamic "Delacor_lib_QMH_Release Message Queue.vi"("error in"=w342, "Message Queue"=w335) -> ("error out"=w341:errorcluster)  [unwired: 9 in]
      n158 = call "Synchronize Caller Events.vi"("Singleton Module Admin in"=w336) -> ("error out"=w343:errorcluster)  [unwired: 9 in, 1 out]
      n159 = call "Module Name--constant.vi"() -> ("Module Name"=w339:string)  [unwired: 11 in]
      n160 = Format Into String(format string="An error occurred during initialization. %s is no longer running.", w339) -> (resulting string=w337:string)  [unwired: 2 in, 1 out]
      n161 = Merge Errors(w341, w343) -> (w344:errorcluster)
      n162 = call "Error Reported.vi"("Additional Information"=w337, "Error"=w344) -> ()  [unwired: 9 in, 1 out]
    }
  }
  n163 = Merge Errors(w14, w17) -> (w13:errorcluster)
  n164 = call "Close Module.vi"("error in"=w13, "Module Admin in"=w8) -> ("error out"=w15:errorcluster, "External Launch"=w2:bool, "Module Admin out"=w3:refnum<class "Delacor_lib_QMH_Module Admin.lvclass">)  [unwired: 7 in]
  n165 = Unregister For Events(event registration refnum=w7, error in=w15) -> (error out=w12:errorcluster)
  "error out" <- w12
  n166 = case "External Launch?" shown="True" w2 {
    tunnel: w12 -> [_ w345]
    frame False {
    }
    frame True {
      n167 = case shown="No Error" w345 {
        frame No Error {
          n168 = invoke on="Invoke Node" class="VI" method="FP.Close"() -> ()  [unwired: 3 in, 3 out]
        }
        frame Error {
          n169 = disable-structure shown="Default" {
            frame condition #0 (active) {
              n170 = invoke class="VI" method="FP.Open"("Activate"=TRUE ("Activate?")) -> ()  [unwired: 4 in, 5 out]
            }
            frame condition #1 {
              # "Don't show panel on error if running inside a built EXE."
            }
          }
        }
      }
    }
  }
  n171 = local write "Module Admin"(w3) -> ()
